vi "Measure_Cap.vi"(8 "error in (no error)":errorcluster, 10 "Parameters":string, 11 "reference in":refnum<class "Test_Flux_Capacitor.lvclass">) -> (0 "error out":errorcluster, 2 "Result":dbl, 3 "reference out":refnum<class "Test_Flux_Capacitor.lvclass">)   [LabVIEW 2022 SP3, in "Test_Flux_Capacitor.lvlib" / "Test_Flux_Capacitor.lvclass"]
uses:
  Test_Flux_Capacitor.lvclass
  ParameterTypes/MeasureCap.ctl
  ParameterTypes/LCR_Meter.ctl
  <vilib>/Utility/error.llb/Trim Whitespace One-Sided.vi
  Components/SwitchBase.lvlibp/SwitchBase.lvclass
  Components/LCR_BK891.lvlibp/LCR_BK891.lvclass
  <vilib>/JDP Science/JSONtext/JSONtext.lvlib
panel:
  in  "Parameter_Type":T1={"Switch"="", "Wait (msec)"=0, "LCR"={"F_(Hz)"=1000.0, "Range"=enum."Auto", "Signal_Level"=enum."0.5Vrms", "Function"=enum."Cp-D", "Meas_Speed"=enum."Fast"}, "Scale"=0.0} {"LCR"."F_(Hz)" format="%#_4g"}
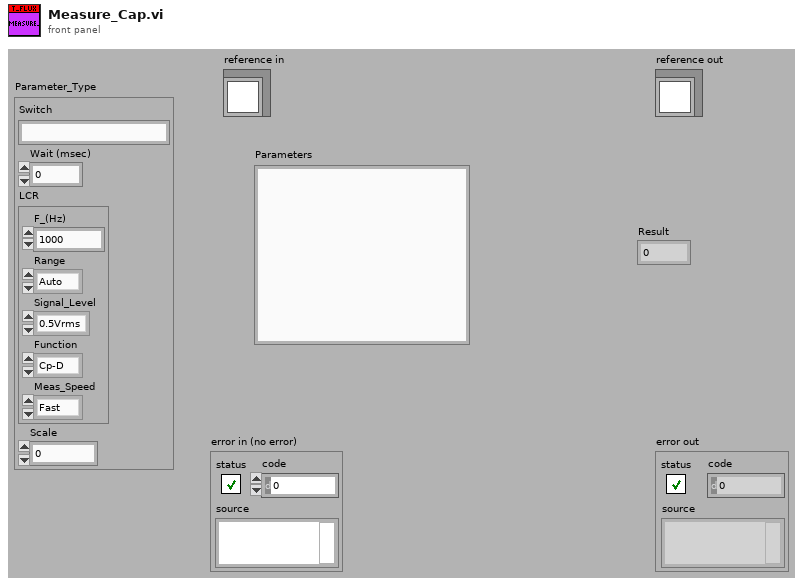
[diagram p1: front panel]
types:
  T1 = typedef "Test_Flux_Capacitor.lvlib/Test_Flux_Capacitor.lvclass/MeasureCap.ctl" = cluster{"Switch":string, "Wait (msec)":u32, "LCR":T2, "Scale":dbl}
  T2 = typedef "Test_Flux_Capacitor.lvlib/Test_Flux_Capacitor.lvclass/LCR_Meter.ctl" = cluster{"F_(Hz)":dbl, "Range":enum16{"Hold", "Auto"}, "Signal_Level":enum16{"0.5Vrms", "1Vrms"}, "Function":enum16{"Cs-Q", "Cs-D", "Cs-R", "Cp-Q", "Cp-D", "Cp-R", "Cp-G", "Ls-Q", "Ls-D", "Ls-R", "Lp-Q", "Lp-D", "Lp-R", "Lp-G", "Z-th", "Y-th", "R-X", "G-B", "DCR"}, "Meas_Speed":enum16{"Slow", "Fast"}}
  T3 = typedef "Test_Flux_Capacitor.lvlib/Test_Flux_Capacitor.lvclass/ObjectAttributes.ctl" = cluster{"Config":T4, "DMM":refnum<class "DMM_Keysight_34980A.lvclass">, "LCR":refnum<class "LCR_BK891.lvclass">, "PSU":refnum<class "PSU_Base.lvclass">, "Switch_Manager":refnum<class "SwitchBase.lvclass">, "FRAM":string, "Flux_Capacitor":refnum<class "Flux_Capacitor.lvclass">, "Frequency_Counter":refnum<class "Frequency_Counter_Base.lvclass">, "JTAG":refnum<class "JTAG_Base.lvclass">}
  T4 = typedef "Test_Flux_Capacitor.lvlib/Test_Flux_Capacitor.lvclass/Config.ctl" = cluster{"default":string}
  T5 = enum16{"Cs-Q", "Cs-D", "Cs-R", "Cp-Q", "Cp-D", "Cp-R", "Cp-G", "Ls-Q", "Ls-D", "Ls-R", "Lp-Q", "Lp-D", "Lp-R", "Lp-G", "Z-th", "Y-th", "R-X", "G-B", "DCR"}
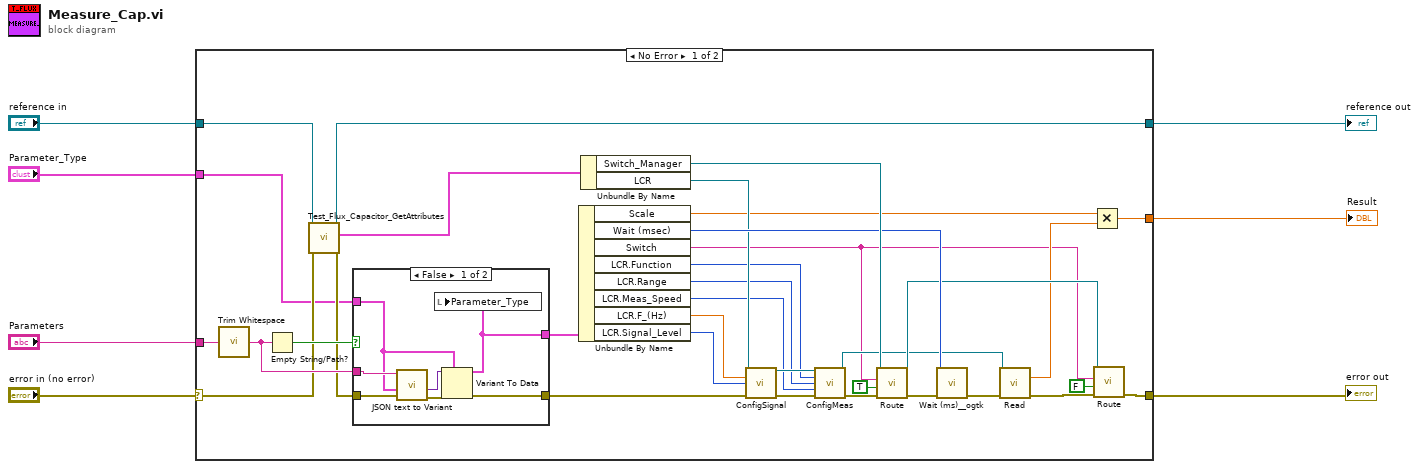
[diagram p0: block diagram]
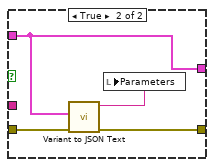
[diagram p2: hidden frame]
diagram:
  n1 = case shown="No Error" "error in (no error)" {
    selector: "error in (no error)" -> [w18 w54]
    tunnel: [w38 w54] -> w6
    tunnel: [w14 w53] -> w4
    tunnel: "reference in" -> [w15 w53]
    tunnel: "Parameters" -> [w16 _]
    tunnel: "Parameter_Type" -> [w12 _]
    tunnel: [w22 _] -> w1
    frame No Error {
      n2 = call <vilib>:"Trim Whitespace.vi"("string"=w16) -> ("trimmed string"=w21:string)  [unwired: 1 in]
      n3 = Empty String/Path?(string/path=w21) -> (empty?=w20:bool)
      n4 = call "Test_Flux_Capacitor_GetAttributes.vi"("error in (no error)"=w18, "reference in"=w15) -> ("error out"=w19:errorcluster, "Data"=w13:T3, "reference out"=w14:refnum<class "Test_Flux_Capacitor.lvclass">)  [unwired: 6 in, 1 out]
      n5 = case shown="False" w20 {
        tunnel: w19 -> [w44 w51]
        tunnel: w12 -> [w45 w52]
        tunnel: [w48 w50] -> w17
        tunnel: [w47 w52] -> w11
        tunnel: w21 -> [w46 _]
        frame False {
          n6 = call <vilib>:"JSON text to Variant.vi"("error in (no error)"=w44, "Data Type"=w45, "JSON"=w46) -> ("error out"=w43:errorcluster, "Variant out"=w42:variant)  [unwired: 7 in]
          n7 = Variant To Data(error in=w43, type=w45, Variant=w42) -> (data=w47:T1, error out=w48:errorcluster)
          n8 = local write "Parameter_Type"(w47) -> ()
        }
        frame True {
          n9 = call <vilib>:"Variant to JSON Text.vi"("error in (no error)"=w51, "Variant"=w52) -> ("error out"=w50:errorcluster, "<JSON>"=w49:string)  [unwired: 7 in, 1 out]
          n10 = local write "Parameters"(w49) -> ()
        }
      }
      n11 = Unbundle By Name(w11) -> ("Scale"=w23:dbl, "Wait (msec)"=w39:u32, "Switch"=w8:string, "LCR.Function"=w30:T5, "LCR.Range"=w29:enum16{"Hold", "Auto"}, "LCR.Meas_Speed"=w28:enum16{"Slow", "Fast"}, "LCR.F_(Hz)"=w36:dbl, "LCR.Signal_Level"=w34:enum16{"0.5Vrms", "1Vrms"})
      n12 = Unbundle By Name(w13) -> ("Switch_Manager"=w41:refnum<class "SwitchBase.lvclass">, "LCR"=w35:refnum<class "LCR_BK891.lvclass">)
      n13 = call-dynamic "ConfigSignal.vi"("reference in"=w35, "Signal Frequency (1000 Hz)"=w36, "Signal Level (0:0.5 Vrms)"=w34, "error in (no error)"=w17) -> ("reference in"=w31:refnum<class "LCR_BK891.lvclass">, "error out"=w33:errorcluster)  [unwired: 10 in]
      n14 = call-dynamic "ConfigMeas.vi"("reference in"=w31, "Function (4: Cp-D)"=w30, "Range (1:Auto)"=w29, "Meas_Speed"=w28, "error in (no error)"=w33) -> ("reference in"=w25:refnum<class "LCR_BK891.lvclass">, "error out"=w32:errorcluster)  [unwired: 9 in]
      n15 = call-dynamic "Route.vi"("error in (no error)"=w32, "Connect"=TRUE, "channel 1"=w8, "reference in"=w41) -> ("error out"=w40:errorcluster, "reference in"=w37:refnum<class "SwitchBase.lvclass">)  [unwired: 6 in]
      n16 = call <userlib>:"Wait (ms)__ogtk.vi"("error in (no error)"=w40, "milliseconds to wait"=w39) -> ("error out"=w27:errorcluster)  [unwired: 8 in, 1 out]
      n17 = call-dynamic "Read.vi"("reference in"=w25, "error in (no error)"=w27) -> ("Measured Primary Reading"=w24:dbl, "error out"=w26:errorcluster)  [unwired: 10 in, 2 out]
      n18 = Multiply(x=w23, y=w24) -> (x*y=w22:dbl)
      n19 = call-dynamic "Route.vi"("error in (no error)"=w26, "Connect"=FALSE, "channel 1"=w8, "reference in"=w37) -> ("error out"=w38:errorcluster)  [unwired: 6 in, 1 out]
    }
    frame Error {
    }
  }
  "Result" <- w1
  "error out" <- w6
  "reference out" <- w4
